vi "Test_Modify_Text_Style.vi"() -> ()   [LabVIEW 2014, in "DSLV_Tree.lvlib"]
uses:
  DSLV_Tree.lvlib
panel:
  in  "Status":string(combo)
  in  "Tree":string(tree)
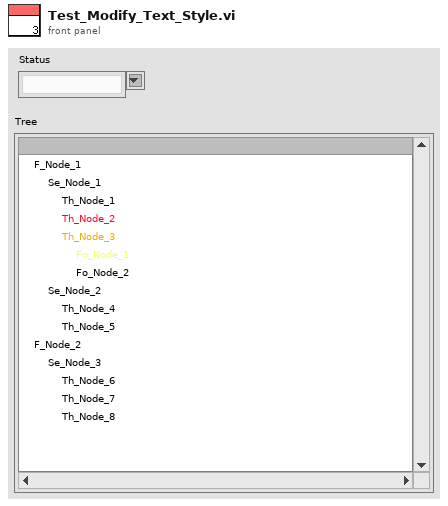
[diagram p1: front panel]
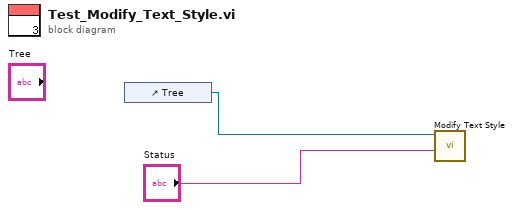
[diagram p0: block diagram]
diagram:
  n1 = control-ref of="Tree"() -> (w2:refnum<vi>)
  n2 = call "Modify Text Style.vi"("Status"="Status", "Tree Reference"=w2) -> ()  [unwired: 8 in, 2 out]
